vi "0-4040_Open232.vi"(8 "error in (no error)":errorcluster, 9 "Flow meter.Units":enum16{"Standard", "Volumetric"}(ring), 10 "baud rate (9600)":u32=38400, 11 "VISA resource name":refnum<visa-resource-name>="COM1") -> (0 "error out":errorcluster, 3 "status":bool)   [LabVIEW 2017]
uses:
  <vilib>/Instr/_visa.llb/VISA Configure Serial Port (Instr).vi
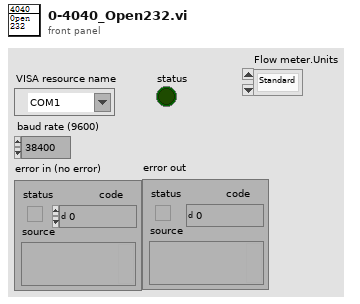
[diagram p1: front panel]
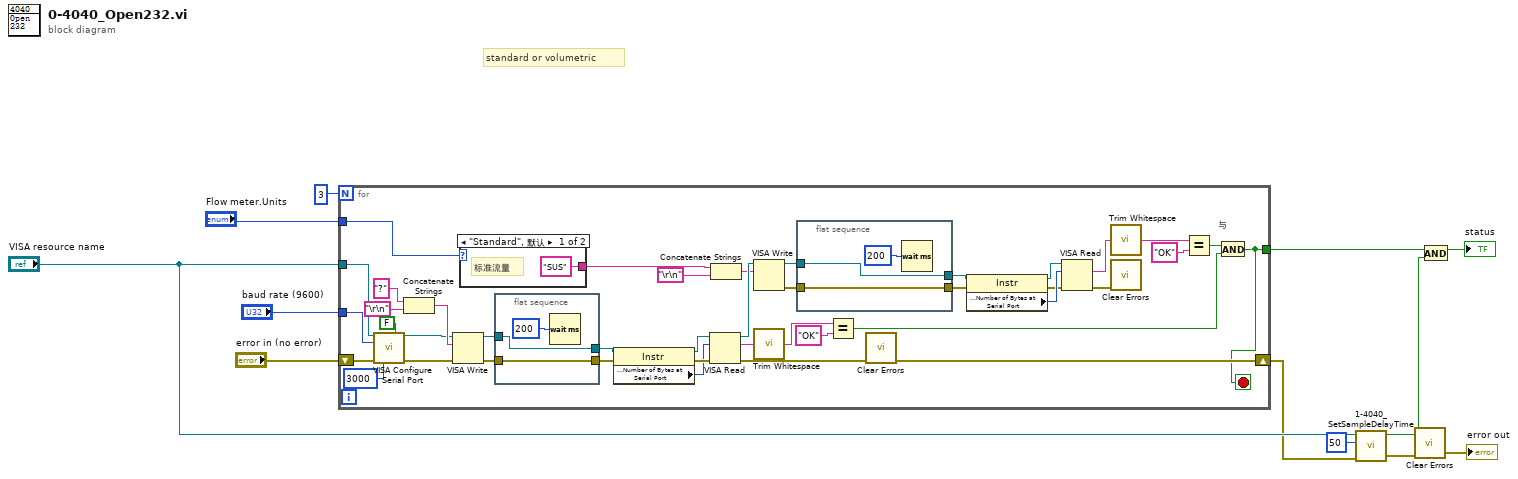
[diagram p0: block diagram]
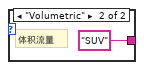
[diagram p2: hidden frame]
diagram:
  # "standard or volumetric"
  n1 = for {
    N: 3 -> [_]
    tunnel: "VISA resource name" -> [w53]
    tunnel: "baud rate (9600)" -> [w52]
    tunnel: [w14] -> w10
    shift-right: [w36] -> w5
    shift-left: "error in (no error)" -> [w51]
    tunnel: "Flow meter.Units" -> [w13]
    stop <- w14 stop-if-true
    n2 = call-poly "VISA Configure Serial Port"("VISA resource name"=w53, "timeout (10sec)"=u32 3000, "Enable Termination\nChar (T)"=FALSE ("Enable Termination\nChar (T)"), "baud rate (9600)"=w52, "error in (no error)"=w51) -> ("VISA resource name out"=w40:refnum<visa-resource-name>, "error out"=w39:errorcluster)  [unwired: 9 in]
    n3 = Concatenate Strings("?" ("写入缓冲区"), "\r\n") -> (w49:string)
    n4 = VISA Write(VISA resource name=w40, write buffer=w49, error in (no error)=w39) -> (VISA resource name out=w38:refnum<visa-resource-name>, error out=w37:errorcluster)  [unwired: 1 out]
    n5 = case shown="\"Standard\", 默认" w13 {
      tunnel: ["SUS" ("写入缓冲区") "SUV" ("写入缓冲区")] -> w15
      frame "Standard", Default {
        # "标准流量"
      }
      frame "Volumetric" {
        # "体积流量"
      }
    }
    n6 = flat-sequence {
      tunnel: w38 -> [w61]
      tunnel: w37 -> [w60]
      tunnel: [w61] -> w32
      tunnel: [w60] -> w33
      frame #0 {
        n7 = Wait (ms)(milliseconds to wait=u32 200) -> ()  [unwired: 1 out]
      }
    }
    n8 = property class="Instr"(reference=w32, error in=w33) -> (reference out=w47:refnum<visa-resource-name>, error out=w46:errorcluster, "Serial Settings:Number of Bytes at Serial Port"=w45:u32)
    n9 = VISA Read(VISA resource name=w47, byte count=w45, error in (no error)=w46) -> (VISA resource name out=w31:refnum<visa-resource-name>, read buffer=w44:string, error out=w41:errorcluster)  [unwired: 1 out]
    n10 = Concatenate Strings(w15, "\r\n") -> (w30:string)
    n11 = VISA Write(VISA resource name=w31, write buffer=w30) -> (VISA resource name out=w29:refnum<visa-resource-name>, error out=w28:errorcluster)  [unwired: 1 in, 1 out]
    n12 = call <vilib>:"Trim Whitespace.vi"("string"=w44) -> ("trimmed string"=w42:string)  [unwired: 1 in]
    n13 = flat-sequence {
      tunnel: w29 -> [w58]
      tunnel: w28 -> [w57]
      tunnel: [w58] -> w22
      tunnel: [w57] -> w21
      frame #0 {
        n14 = Wait (ms)(milliseconds to wait=u32 200) -> ()  [unwired: 1 out]
      }
    }
    n15 = Equal?(x=w42, y="OK") -> (x = y?=w35:bool)
    n16 = call <vilib>:"Clear Errors.vi"("error in (no error)"=w41) -> ("error out"=w36:errorcluster)  [unwired: 5 in, 1 out]
    n17 = property class="Instr"(reference=w22, error in=w21) -> (reference out=w23:refnum<visa-resource-name>, error out=w24:errorcluster, "Serial Settings:Number of Bytes at Serial Port"=w25:u32)
    n18 = VISA Read(VISA resource name=w23, byte count=w25, error in (no error)=w24) -> (read buffer=w26:string, error out=w27:errorcluster)  [unwired: 2 out]
    n19 = call <vilib>:"Trim Whitespace.vi"("string"=w26) -> ("trimmed string"=w19:string)  [unwired: 1 in]
    n20 = call <vilib>:"Clear Errors.vi"("error in (no error)"=w27) -> ()  [unwired: 5 in, 2 out]
    n21 = Equal?(x=w19, y="OK") -> (x = y?=w18:bool)
    n22 = And "与"(x=w18, y=w35) -> (x .and. y?=w14:bool)
  }
  n23 = call "1-4040_SetSampleDelayTime.vi"("Error in"=w5, "Sample Delay Time(ms)"=50, "Visa IO"="VISA resource name") -> ("error out"=w2:errorcluster, "SetSuccessful?"=w3:bool)  [unwired: 7 in]
  n24 = call <vilib>:"Clear Errors.vi"("error in (no error)"=w2) -> ("error out"=→"error out":errorcluster)  [unwired: 5 in, 1 out]
  n25 = And(x=w10, y=w3) -> (x .and. y?=→"status":bool)
